vi "MIDI-Generator.vi"() -> ()   [LabVIEW 2019]
uses:
  Controls/Generator_states.ctl
panel:
  in  "Clear":bool
  in  "Save":bool
  in  "Name of message":string
  out "MIDI Events":string
  in  "Last Nibble":u16(ring)
  out "Databyte 2":i8 format="%.0x"
  out "Databyte 1":i8 format="%.0x"
  in  "Spec Concatenate":bool
  out "MIDI Event":string
  in  "Databyte 2":u16(ring) caption="Pressure" items=["0", "1", "2", "3", "4", "5", "6", "7", "8", "9", "10", "11", "12", "13", "14", "15", "16", "17", "18", "19", "20", "21", "22", "23", "24", "25", "26", "27", "28", "29", "30", "31", "32", "33", "34", "35", "36", "37", "38", "39", "40", "41", "42", "43", "44", "45", "46", "47", "48", "49", "50", "51", "52", "53", "54", "55", "56", "57", "58", "59", "60", "61", "62", "63", "64", "65", "66", "67", "68", "69", "70", "71", "72", "73", "74", "75", "76", "77", "78", "79", "80", "81", "82", "83", "84", "85", "86", "87", "88", "89", "90", "91", "92", "93", "94", "95", "96", "97", "98", "99", "100", "101", "102", "103", "104", "105", "106", "107", "108", "109", "110", "111", "112", "113", "114", "115", "116", "117", "118", "119", "120", "121", "122", "123", "124", "125", "126", "127"]
  in  "Databyte 1":u16(ring) caption="Note #" items=["C-1", "C#-1", "D-1", "D#-1", "E-1", "F-1", "F#-1", "G-1", "G#-1", "A-1", "A#-1", "B-1", "C0", "C#0", "D0", "D#0", "E0", "F0", "F#0", "G0", "G#0", "A0", "A#0", "B0", "C1", "C#1", "D1", "D#1", "E1", "F1", "F#1", "G1", "G#1", "A1", "A#1", "B1", "C2", "C#2", "D2", "D#2", "E2", "F2", "F#2", "G2", "G#2", "A2", "A#2", "B2", "C3", "C#3", "D3", "D#3", "E3", "F3", "F#3", "G3", "G#3", "A3", "A#3", "B3", "C4", "C#4", "D4", "D#4", "E4", "F4", "F#4", "G4", "G#4", "A4", "A#4", "B4", "C5", "C#5", "D5", "D#5", "E5", "F5", "F#5", "G5", "G#5", "A5", "A#5", "B5", "C6", "C#6", "D6", "D#6", "E6", "F6", "F#6", "G6", "G#6", "A6", "A#6", "B6", "C7", "C#7", "D7", "D#7", "E7", "F7", "F#7", "G7", "G#7", "A7", "A#7", "B7", "C8", "C#8", "D8", "D#8", "E8", "F8", "F#8", "G8", "G#8", "A8", "A#8", "B8", "C9", "C#9", "D9", "D#9", "E9", "F9", "F#9", "G9"]
  in  "2. Nibble":u8(ring) caption="Channel" items=["Channel 1", "Channel 2", "Channel 3", "Channel 4", "Channel 5", "Channel 6", "Channel 7", "Channel 8", "Channel 9", "Channel 10", "Channel 11", "Channel 12", "Channel 13", "Channel 14", "Channel 15", "Channel 16"]
  out "Statusbyte":i8 format="%.0x"
  in  "Status":T1(ring)
  # "Spec Concatenation"
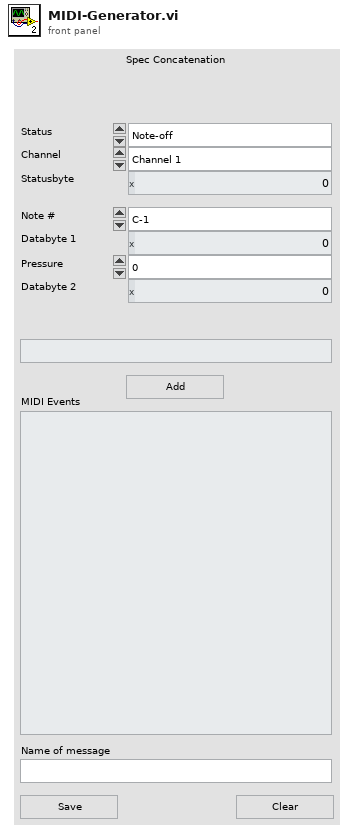
[diagram p1: front panel]
types:
  T1 = enum16{"Note-off", "Note-on", "Polyphonic Key Pressure (aftertouch)", "Control Change", "Program Change", "Channel Pressure (After-Touch)", "Pitch Bend Change", "System Common msg"}
  T2 = typedef "Generator_states.ctl" = enum16{"Initiate", "Wait for event", "Prep 2nd Nibble", "Prep Databyte 1", "Parse Databyte 1", "Prep Databyte 2", "Parse Databyte 2", "Print Event", "Save MIDI Event", "Generate Function", "Save as Textfile"}
  T3 = cluster{"1st Nibble":enum16{"Note-off", "Note-on", "Polyphonic Key Pressure (aftertouch)", "Control Change", "Program Change", "Channel Pressure (After-Touch)", "Pitch Bend Change", "System Common msg"}, "Next state":T2, "2nd Nibble":u8, "Databyte 1":u16, "Keep 2nd Nibble":bool, "Databyte 2":i32, "Last Nibble":u16, "MIDI Event":string, "MIDI Events":string}
  T4 = enum16{"open", "replace", "create", "open or create", "replace or create", "replace or create with confirmation"}
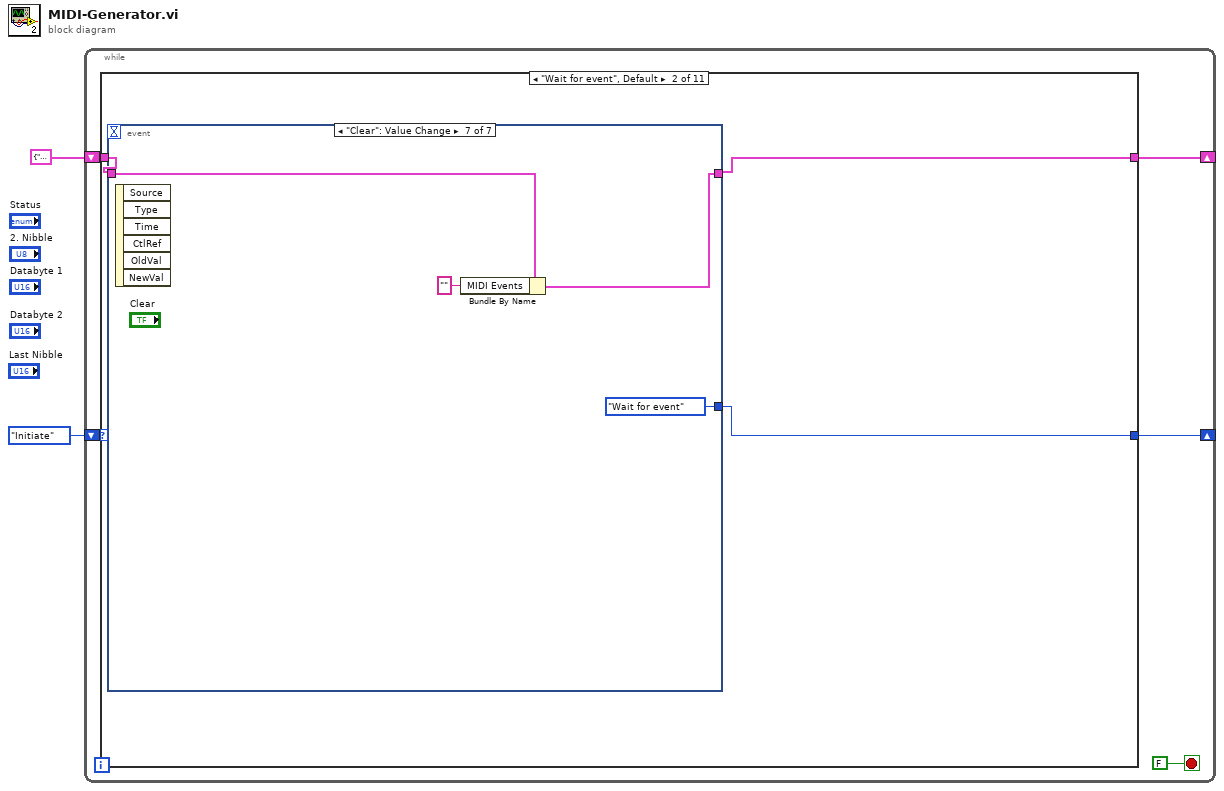
[diagram p0: block diagram]
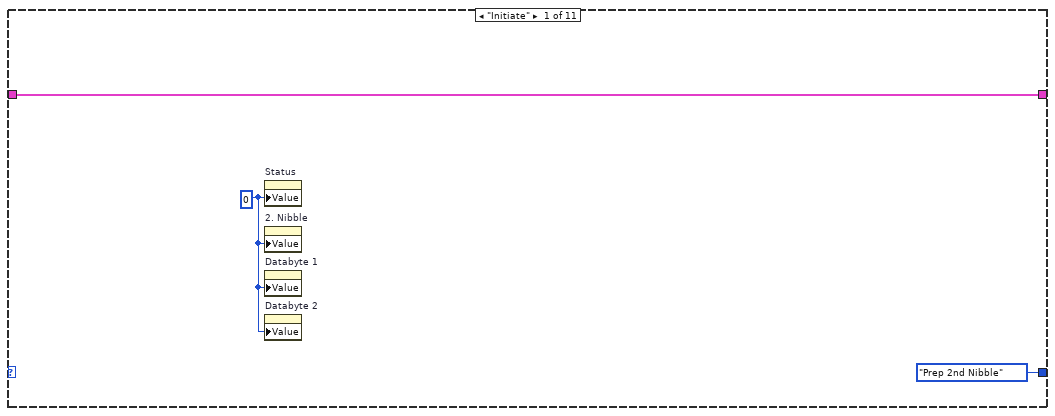
[diagram p2: hidden frame]
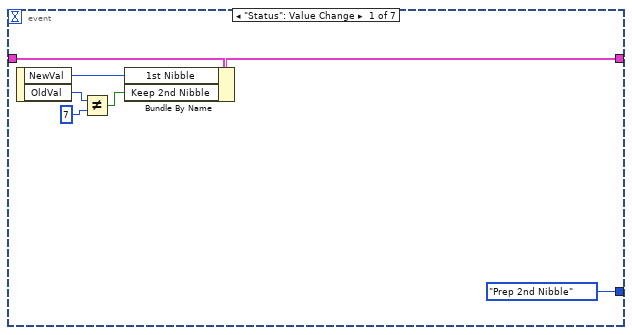
[diagram p3: hidden frame]
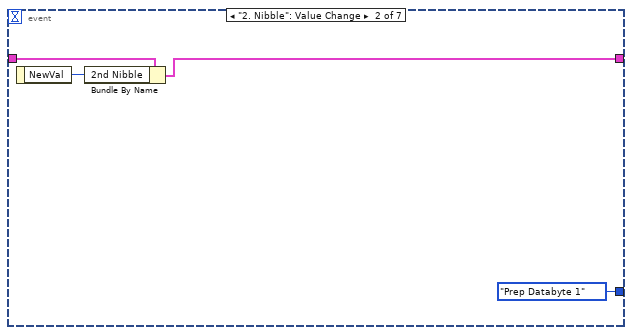
[diagram p4: hidden frame]
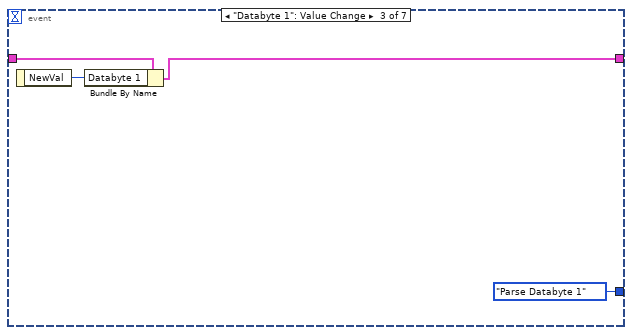
[diagram p5: hidden frame]
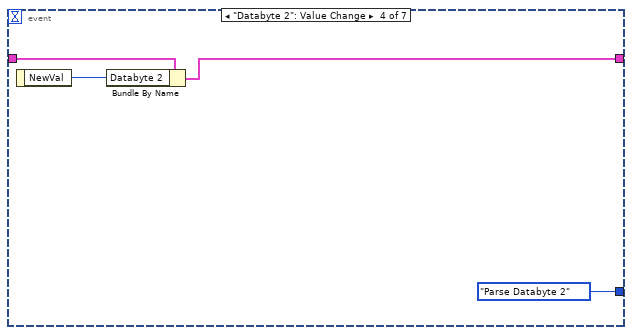
[diagram p6: hidden frame]
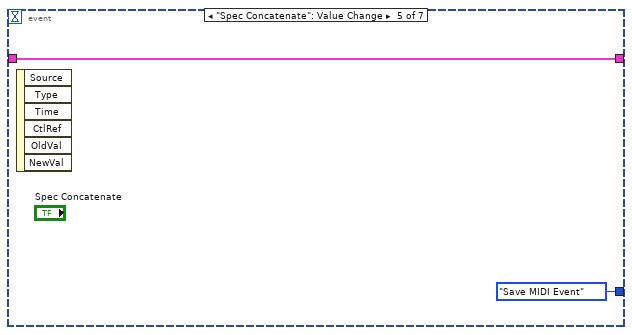
[diagram p7: hidden frame]
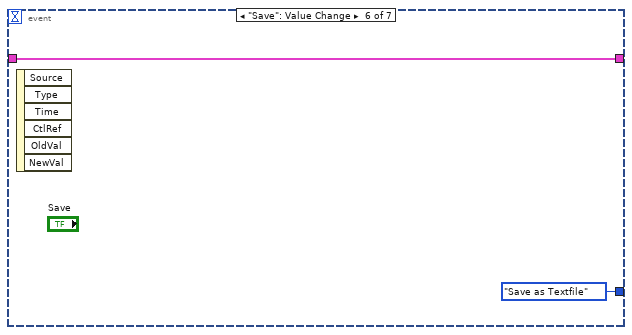
[diagram p8: hidden frame]
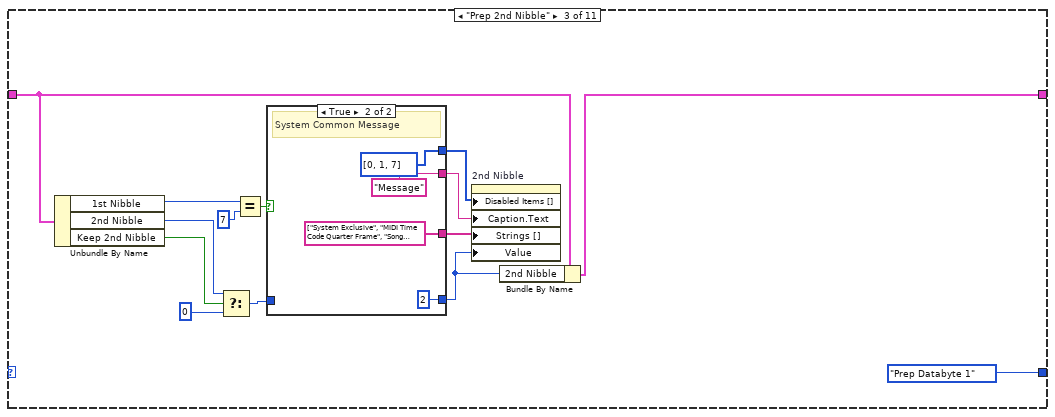
[diagram p9: hidden frame]
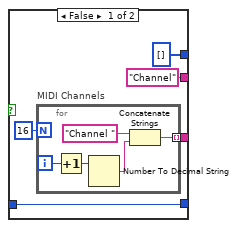
[diagram p10: hidden frame]
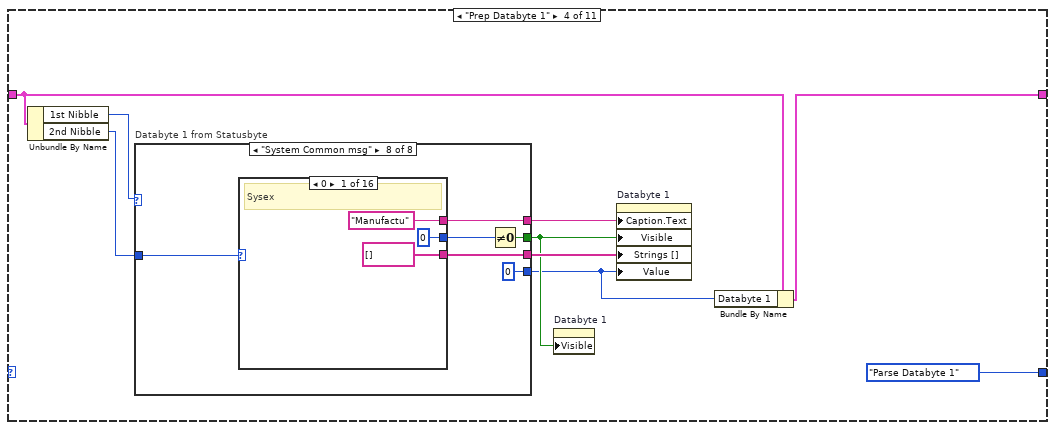
[diagram p11: hidden frame]
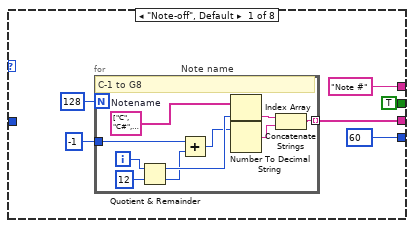
[diagram p12: hidden frame]
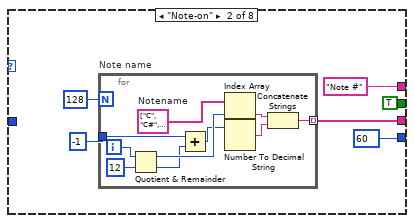
[diagram p13: hidden frame]
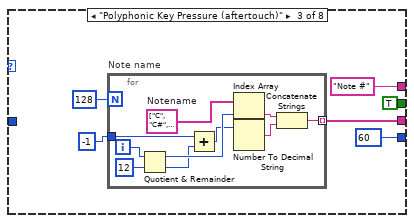
[diagram p14: hidden frame]
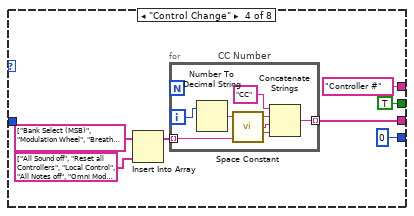
[diagram p15: hidden frame]
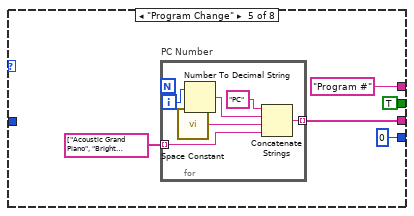
[diagram p16: hidden frame]
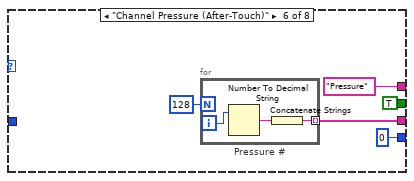
[diagram p17: hidden frame]
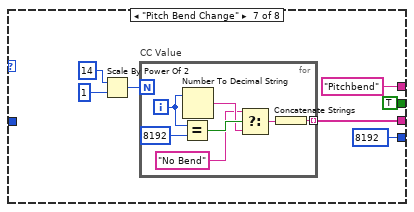
[diagram p18: hidden frame]
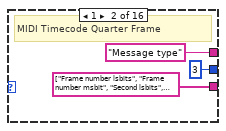
[diagram p19: hidden frame]
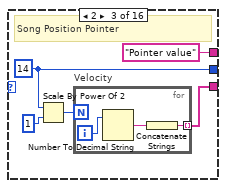
[diagram p20: hidden frame]
diagram:
  n1 = while {
    shift-right: [w3] -> _
    shift-left: T3 {"1st Nibble"=enum."Note-off", "Next state"=enum."Wait for event", "2nd Nibble"=0, "Databyte 1"=0, "Keep 2nd Nibble"=TRUE, "Databyte 2"=241, "Last Nibble"=0, "MIDI Event"="", "MIDI Events"=""} -> [w7]
    shift-right: [w4] -> _
    shift-left: Generator_states."Initiate" ("Status 2") -> [w6]
    stop <- FALSE stop-if-true
    n2 = case shown="\"Wait for event\", Default" w6 {
      tunnel: w7 -> [w10 w13 w43 w71 w239 w290 w566 w603 w621 w625 w636]
      tunnel: [w10 w12 w41 w70 w238 w288 w564 w602 w619 w625 w636] -> w3
      tunnel: [Generator_states."Prep 2nd Nibble" ("Status 2") w11 Generator_states."Prep Databyte 1" ("Status 2") Generator_states."Parse Databyte 1" ("Status 2") Generator_states."Prep Databyte 2" ("Status 2") Generator_states."Parse Databyte 2" ("Status 2") Generator_states."Print Event" ("Status 2") Generator_states."Wait for event" ("Status 2") Generator_states."Wait for event" ("Status 2") Generator_states."Wait for event" ("Status 2") Generator_states."Wait for event" ("Status 2")] -> w4
      frame "Initiate" {
        w9 = 0
        n3 = property on="Status" class="Enum (strict)"("Value"=w9) -> ()  [unwired: 2 in, 2 out]
        n4 = property on="2. Nibble" class="Ring (strict)"("Value"=w9) -> ()  [unwired: 2 in, 2 out]
        n5 = property on="Databyte 1" class="Ring (strict)"("Value"=w9) -> ()  [unwired: 2 in, 2 out]
        n6 = property on="Databyte 2" class="Ring (strict)"("Value"=w9) -> ()  [unwired: 2 in, 2 out]
      }
      frame "Wait for event", Default {
        n7 = event shown="[6] \"Clear\": Value Change" {
          selector: _ -> [_ _ _ _ _ _ _]
          dyn-events: _ -> [_ _ _ _ _ _ _]
          timeout: _ -> [_ _ _ _ _ _ _]
          tunnel: [w18 w21 w25 w30 w34 w36 w39] -> w12
          tunnel: w13 -> [w20 w23 w26 w31 w34 w36 w40]
          tunnel: [Generator_states."Prep 2nd Nibble" ("Status 2") Generator_states."Prep Databyte 1" ("Status 2") Generator_states."Parse Databyte 1" ("Status 2") Generator_states."Parse Databyte 2" ("Status 2") Generator_states."Save MIDI Event" ("Status 2") Generator_states."Save as Textfile" ("Status 2") Generator_states."Wait for event" ("Status 2")] -> w11
          event "Status": Value Change {
            n8 = event-data() -> ("NewVal"=w19:T1, "OldVal"=w16:T1)  [unwired: 1 in]
            n9 = Not Equal?(x=w16, y=7) -> (x != y?=w14:bool)
            n10 = Bundle By Name(cluster=w20, "1st Nibble"=w19, "Keep 2nd Nibble"=w14) -> (w18:T3)
          }
          event "2. Nibble": Value Change {
            n11 = event-data() -> ("NewVal"=w22:u8)  [unwired: 1 in]
            n12 = Bundle By Name(cluster=w23, "2nd Nibble"=w22) -> (w21:T3)
          }
          event "Databyte 1": Value Change {
            n13 = event-data() -> ("NewVal"=w27:u16)  [unwired: 1 in]
            n14 = Bundle By Name(cluster=w26, "Databyte 1"=w27) -> (w25:T3)
          }
          event "Databyte 2": Value Change {
            n15 = event-data() -> ("NewVal"=w32:u16)  [unwired: 1 in]
            n16 = Bundle By Name(cluster=w31, "Databyte 2"=w32) -> (w30:T3)
          }
          event "Spec Concatenate": Value Change {
            n17 = event-data() -> ()  [unwired: 1 in, 6 out]
          }
          event "Save": Value Change {
            n18 = event-data() -> ()  [unwired: 1 in, 6 out]
          }
          event "Clear": Value Change {
            n19 = event-data() -> ()  [unwired: 1 in, 6 out]
            n20 = Bundle By Name(cluster=w40, "MIDI Events"="") -> (w39:T3)
          }
        }
      }
      frame "Prep 2nd Nibble" {
        n21 = Unbundle By Name(w43) -> ("1st Nibble"=w49:T1, "2nd Nibble"=w46:u8, "Keep 2nd Nibble"=w47:bool)
        n22 = Select(t=w46, s=w47, f=u8 0) -> (s? t:f=w45:u8)
        n23 = Equal?(x=w49, y=7) -> (x = y?=w54:bool)
        n24 = case shown="True" w54 {
          tunnel: [w58 string[] ["System Exclusive", "MIDI Time Code Quarter Frame", "Song Position Pointer", "Song Select", "Undefined (Reserved) 1", "Undefined (Reserved) 2", "Tune Request", "End of Exclusive", "Timing Clock", "Undefined (Reserved) 3", "Start", "Continue", "Stop", "Undefined (Reserved) 4", "Active Sensing", "Reset"] ("System Common Messages")] -> w51
          tunnel: ["Channel" "Message" ("t")] -> w52
          tunnel: [i32[] [] ("Disabled Items []") i32[] [0, 1, 7] ("Disabled Items []")] -> w53
          tunnel: [w55 2] -> w42
          tunnel: w45 -> [w55 _]
          frame False {
            n25 = for "MIDI Channels" {
              N: 16 -> [_]
              tunnel: [w61] -> w58 mode=indexing
              i -> [w64]
              n26 = Increment(x=w64) -> (x+1=w60:i32)
              n27 = Number To Decimal String(number=w60) -> (decimal integer string=w63:string)  [unwired: 1 in]
              n28 = Concatenate Strings("Channel " ("string"), w63) -> (w61:string)
            }
          }
          frame True {
            # "System Common Message"
          }
        }
        n29 = property on="2nd Nibble" class="Ring (strict)"("Disabled Items []"=w53, "Caption.Text"=w52, "Strings []"=w51, "Value"=w42) -> ()  [unwired: 2 in, 2 out]
        n30 = Bundle By Name(cluster=w43, "2nd Nibble"=w42) -> (w41:T3)
      }
      frame "Prep Databyte 1" {
        n31 = Unbundle By Name(w71) -> ("1st Nibble"=w74:T1, "2nd Nibble"=w73:u8)
        n32 = case "Databyte 1 from Statusbyte" shown="\"System Common msg\"" w74 {
          tunnel: ["Note #" "Note #" "Note #" "Controller #" "Program #" "Pressure" "Pitchbend" w175] -> w75
          tunnel: [w79 w95 w111 w129 w140 w152 w160 w174] -> w76
          tunnel: [TRUE TRUE TRUE TRUE TRUE TRUE TRUE w177] -> w72
          tunnel: w73 -> [_ _ _ _ _ _ _ w173]
          tunnel: [60 60 60 0 0 0 8192 0] -> w69
          frame "Note-off", Default {
            n33 = for "Note name" {
              N: 128 -> [_]
              tunnel: -1 -> [w89]
              tunnel: [w84] -> w79 mode=indexing
              i -> [w92]
              w93 = string[] ["C", "C#", "D", "D#", "E", "F", "F#", "G", "G#", "A", "A#", "B"]  # Notename
              # "C-1 to G8"
              n34 = Quotient & Remainder(x=w92, y=12) -> (x-y*floor(x/y)=w90:i32, floor(x/y)=w88:i32)
              n35 = Add(x=w89, y=w88) -> (x+y=w87:i32)
              n36 = Index Array(array=w93, index=w90) -> (element=w85:string)
              n37 = Number To Decimal String(number=w87) -> (decimal integer string=w86:string)  [unwired: 1 in]
              n38 = Concatenate Strings(w85, w86) -> (w84:string)
            }
          }
          frame "Note-on" {
            n39 = for "Note name" {
              N: 128 -> [_]
              tunnel: -1 -> [w105]
              tunnel: [w100] -> w95 mode=indexing
              i -> [w108]
              w109 = string[] ["C", "C#", "D", "D#", "E", "F", "F#", "G", "G#", "A", "A#", "B"]  # Notename
              n40 = Quotient & Remainder(x=w108, y=12) -> (x-y*floor(x/y)=w106:i32, floor(x/y)=w104:i32)
              n41 = Add(x=w105, y=w104) -> (x+y=w103:i32)
              n42 = Index Array(array=w109, index=w106) -> (element=w101:string)
              n43 = Number To Decimal String(number=w103) -> (decimal integer string=w102:string)  [unwired: 1 in]
              n44 = Concatenate Strings(w101, w102) -> (w100:string)
            }
          }
          frame "Polyphonic Key Pressure (aftertouch)" {
            n45 = for "Note name" {
              N: 128 -> [_]
              tunnel: -1 -> [w121]
              tunnel: [w116] -> w111 mode=indexing
              i -> [w124]
              w125 = string[] ["C", "C#", "D", "D#", "E", "F", "F#", "G", "G#", "A", "A#", "B"]  # Notename
              n46 = Quotient & Remainder(x=w124, y=12) -> (x-y*floor(x/y)=w122:i32, floor(x/y)=w120:i32)
              n47 = Add(x=w121, y=w120) -> (x+y=w119:i32)
              n48 = Index Array(array=w125, index=w122) -> (element=w117:string)
              n49 = Number To Decimal String(number=w119) -> (decimal integer string=w118:string)  [unwired: 1 in]
              n50 = Concatenate Strings(w117, w118) -> (w116:string)
            }
          }
          frame "Control Change" {
            n51 = Insert Into Array(array=string[] ["Bank Select (MSB)", "Modulation Wheel", "Breath controller", "Undefined", "Foot Pedal (MSB)", "Portamento Time (MSB)", "Data Entry (MSB)", "Volume (MSB)", "Balance (MSB", "Undefined", "Pan position (MSB)", "Expression (MSB)", "Effect Control 1 (MSB)", "Effect Control 2 (MSB)", "Undefined", "Undefined", "General Purpose", "General Purpose", "General Purpose", "General Purpose", "Undefined", "Undefined", "Undefined", "Undefined", "Undefined", "Undefined", "Undefined", "Undefined", "Undefined", "Undefined", "Undefined", "Undefined", "Controller 0", "Controller 1", "Controller 2", "Controller 3", "Controller 4", "Controller 5", "Controller 6", "Controller 7", "Controller 8", "Controller 9", "Controller 10", "Controller 11", "Controller 12", "Controller 13", "Controller 14", "Controller 15", "Controller 16", "Controller 17", "Controller 18", "Controller 19", "Controller 20", "Controller 21", "Controller 22", "Controller 23", "Controller 24", "Controller 25", "Controller 26", "Controller 27", "Controller 28", "Controller 29", "Controller 30", "Controller 31", "Hold Pedal (on/off)", "Portamento (on/off)", "Sostenuto Pedal (on/off)", "Soft Pedal (on/off)", "Legato Pedal (on/off)", "Hold 2 Pedal (on/off)", "Sound Variation", "Resonance (Timbre)", "Sound Release Time", "Sound Attack Time", "Frequency Cutoff (Brightness)", "Sound Control 6", "Sound Control 7", "Sound Control 8", "Sound Control 9", "Sound Control 10", "Decay or General Purpose Button 1 (on/off) Roland Tone level 1", "Hi Pass Filter Frequency or General Purpose Button 2 (on/off) Roland Tone level 2", "General Purpose Button 3 (on/off) Roland Tone level 3", "General Purpose Button 4 (on/off) Roland Tone level 4", "Portamento Amount", "Undefined", "Undefined", "Undefined", "Undefined", "Undefined", "Undefined", "Reverb Level", "Tremolo Level", "Chorus Level", "Detune Level", "Phaser Level", "Data Button increment", "Data Button decrement", "Non-registered Parameter (LSB)", "Non-registered Parameter (MSB)", "Registered Parameter (LSB)", "Registered Parameter (MSB)", "Undefined", "Undefined", "Undefined", "Undefined", "Undefined", "Undefined", "Undefined", "Undefined", "Undefined", "Undefined", "Undefined", "Undefined", "Undefined", "Undefined", "Undefined", "Undefined", "Undefined", "Undefined"], new element=string[] ["All Sound off", "Reset all Controllers", "Local Control", "All Notes off", "Omni Mode off", "Omni Mode on", "Mono Mode", "Poly Mode"]) -> (w127:string[])  [unwired: 1 in]
            n52 = for "CC Number" {
              tunnel: [w136] -> w129 mode=indexing
              tunnel: w127 -> [w133] mode=indexing
              i -> [w135]
              n53 = Number To Decimal String(number=w135) -> (decimal integer string=w138:string)  [unwired: 1 in]
              n54 = call <vilib>:"Space Constant.vi"() -> ("String"=w134:string)
              n55 = Concatenate Strings("CC" ("string"), w138, w134, w133) -> (w136:string)
            }
          }
          frame "Program Change" {
            n56 = for "PC Number" {
              tunnel: [w146] -> w140 mode=indexing
              tunnel: string[] ["Acoustic Grand Piano", "Bright Acoustic Piano", "Electric Grand Piano", "Honky-tonk Piano", "Electric Piano 1", "Electric Piano 2", "Harpsichord", "Clavinet", "Celesta", "Glockenspiel", "Music Box", "Vibraphone", "Marimba", "Xylophone", "Tubular Bells", "Dulcimer", "Drawbar Organ", "Percussive Organ", "Rock Organ", "Church Organ", "Reed Organ", "Accordion", "Harmonica", "Tango accordion", "Acoustic Guitar (nylon)", "Acoustic Guitar (steel)", "Electric Guitar (jazz)", "Electric Guitar (clean)", "Electric Guitar (muted)", "Overdriven Guitar", "Distortion Guitar", "Guitar Harmonics", "Acoustic Bass", "Electric Bass (finger)", "Electric Bass (pick)", "Fretless Bass", "Slap Bass 1", "Slap Bass 2", "Synth Bass 1", "Synth Bass 2", "Violin", "Viola", "Cello", "Contrabass", "Tremolo Strings", "Pizzicato Strings", "Orchestral Harp", "Timpani", "String Ensemble 1", "String Ensemble 2", "Synth Strings 1", "Synth Strings 2", "Choir Aahs", "Voice Oohs", "Synth Choir", "Orchestra Hit", "Trumpet", "Trombone", "Tuba", "Muted Trumpet", "French Horn", "Brass Section", "Synth Brass 1", "Synth Brass 2", "Soprano Sax", "Alto Sax", "Tenor Sax", "Baritone Sax", "Oboe", "English Horn", "Bassoon", "Clarinet", "Piccolo", "Flute", "Recorder", "Pan Flute", "Blown bottle", "Shakuhachi", "Whistle", "Ocarina", "Lead 1 (square)", "Lead 2 (sawtooth)", "Lead 3 (calliope)", "Lead 4 (chiff)", "Lead 5 (charang)", "Lead 6 (voice)", "Lead 7 (fifths)", "Lead 8 (bass + lead)", "Pad 1 (new age)", "Pad 2 (warm)", "Pad 3 (polysynth)", "Pad 4 (choir)", "Pad 5 (bowed)", "Pad 6 (metallic)", "Pad 7 (halo)", "Pad 8 (sweep)", "FX 1 (rain)", "FX 2 (soundtrack)", "FX 3 (crystal)", "FX 4 (atmosphere)", "FX 5 (brightness)", "FX 6 (goblins)", "FX 7 (echoes)", "FX 8 (sci-fi)", "Sitar", "Banjo", "Shamisen", "Koto", "Kalimba", "Bagpipe", "Fiddle", "Shanai", "Tinkle Bell", "Agogo", "Steel Drums", "Woodblock", "Taiko Drum", "Melodic Tom", "Synth Drum", "Reverse Cymbal", "Guitar Fret Noise", "Breath Noise", "Seashore", "Bird Tweet", "Telephone Ring", "Helicopter", "Applause", "Gunshot", "??"] -> [w144] mode=indexing
              i -> [w149]
              n57 = call <vilib>:"Space Constant.vi"() -> ("String"=w145:string)
              n58 = Number To Decimal String(number=w149) -> (decimal integer string=w148:string)  [unwired: 1 in]
              n59 = Concatenate Strings("PC" ("string"), w148, w145, w144) -> (w146:string)
            }
          }
          frame "Channel Pressure (After-Touch)" {
            n60 = for "Pressure #" {
              N: 128 -> [_]
              tunnel: [w156] -> w152 mode=indexing
              i -> [w155]
              n61 = Number To Decimal String(number=w155) -> (decimal integer string=w157:string)  [unwired: 1 in]
              n62 = Concatenate Strings(w157) -> (w156:string)
            }
          }
          frame "Pitch Bend Change" {
            n63 = Scale By Power Of 2(n=i16 14, x=i16 1 ("n")) -> (x*2^n=w159:i16)
            n64 = for "CC Value" {
              N: w159 -> [_]
              tunnel: [w171] -> w160 mode=indexing
              i -> [w169]
              n65 = Equal?(x=w169, y=8192) -> (x = y?=w170:bool)
              n66 = Number To Decimal String(number=w169) -> (decimal integer string=w166:string)  [unwired: 1 in]
              n67 = Select(t="No Bend", s=w170, f=w166) -> (s? t:f=w167:string)
              n68 = Concatenate Strings(w167) -> (w171:string)
            }
          }
          frame "System Common msg" {
            n69 = case shown="0" w173 {
              tunnel: ["Manufactu" "Message type" "Pointer value" "Sequence" "" "" "" "" "" "" "" "" "" "" "" ""] -> w175
              tunnel: [string[] [] string[] ["Frame number lsbits", "Frame number msbit", "Second lsbits", "Second msbits", "Minute lsbits", "Minute msbits", "Hour lsbits", "Rate and hour msbit"] w185 w193 string[] [] string[] [] string[] [] string[] [] string[] [] string[] [] string[] [] string[] [] string[] [] string[] [] string[] [] string[] []] -> w174
              tunnel: [0 3 w186 w194 0 0 0 0 0 0 0 0 0 0 0 0] -> w176
              frame 0 {
                # "Sysex"
              }
              frame 1 {
                # "MIDI Timecode Quarter Frame"
              }
              frame 2 {
                w186 = 14
                # "Song Position Pointer"
                n70 = Scale By Power Of 2(n=w186, x=1) -> (x*2^n=w184:i32)
                n71 = for "Velocity" {
                  N: w184 -> [_]
                  tunnel: [w190] -> w185 mode=indexing
                  i -> [w189]
                  n72 = Number To Decimal String(number=w189) -> (decimal integer string=w191:string)  [unwired: 1 in]
                  n73 = Concatenate Strings(w191) -> (w190:string)
                }
              }
              frame 3 {
                w194 = 7
                # "Song Select"
                n74 = Scale By Power Of 2(n=w194, x=1) -> (x*2^n=w192:i32)
                n75 = for "Velocity" {
                  N: w192 -> [_]
                  tunnel: [w198] -> w193 mode=indexing
                  i -> [w197]
                  n76 = Number To Decimal String(number=w197) -> (decimal integer string=w199:string)  [unwired: 1 in]
                  n77 = Concatenate Strings(w199) -> (w198:string)
                }
              }
              frame 4, Default {
                # "Undefined 1"
              }
              frame 5 {
                # "Undefined 2"
              }
              frame 6 {
                # "Tune Request"
              }
              frame 7 {
                # "End of Exclusive"
              }
              frame 8 {
                # "Timing Clock"
              }
              frame 9 {
                # "Undefined 3"
              }
              frame 10 {
                # "Start"
              }
              frame 11 {
                # "Continue"
              }
              frame 12 {
                # "Stop"
              }
              frame 13 {
                # "Undefined 4"
              }
              frame 14 {
                # "Active Sensing"
              }
              frame 15 {
                # "Reset"
              }
            }
            n78 = Not Equal To 0?(x=w176) -> (x != 0?=w177:bool)
          }
        }
        n79 = property on="Databyte 1" class="DigNum (strict)"("Visible"=w72) -> ()  [unwired: 2 in, 2 out]
        n80 = property on="Databyte 1" class="Ring (strict)"("Caption.Text"=w75, "Visible"=w72, "Strings []"=w76, "Value"=w69) -> ()  [unwired: 2 in, 2 out]
        n81 = Bundle By Name(cluster=w71, "Databyte 1"=w69) -> (w70:T3)
      }
      frame "Parse Databyte 1" {
        n82 = Unbundle By Name(w239) -> ("1st Nibble"=w241:T1, "2nd Nibble"=w237:u8, "Databyte 1"=w240:u16)
        n83 = case shown="\"System Common msg\"" w241 {
          tunnel: w240 -> [_ _ _ _ _ _ w252 w254]
          tunnel: w239 -> [w242 w243 w244 w245 w246 w247 w251 w257]
          tunnel: [w242 w243 w244 w245 w246 w247 w250 w256] -> w238
          tunnel: w237 -> [_ _ _ _ _ _ _ w255]
          frame "Note-off", Default {
          }
          frame "Note-on" {
          }
          frame "Polyphonic Key Pressure (aftertouch)" {
          }
          frame "Control Change" {
          }
          frame "Program Change" {
          }
          frame "Channel Pressure (After-Touch)" {
          }
          frame "Pitch Bend Change" {
            n84 = Rotate(1:w252, 2:i16 -7 ("y 2")) -> (0:w248:u16)
            n85 = Subtract(x=w252, y=w248) -> (x-y=w249:u16)
            n86 = Bundle By Name(cluster=w251, "Databyte 2"=w249, "Databyte 1"=w248) -> (w250:T3)
          }
          frame "System Common msg" {
            n87 = case shown="1" w255 {
              tunnel: w257 -> [w258 w259 w264 w268 w269 w270 w271 w272 w273 w274 w275 w276 w277 w278 w279 w280]
              tunnel: [w258 w259 w265 w267 w269 w270 w271 w272 w273 w274 w275 w276 w277 w278 w279 w280] -> w256
              tunnel: w254 -> [_ _ w262 w266 _ _ _ _ _ _ _ _ _ _ _ _]
              frame 0 {
                # "Sysex"
              }
              frame 1 {
                # "MIDI Timecode Quarter Frame"
              }
              frame 2 {
                # "Song Position Pointer"
                n88 = Rotate(1:w262, 2:i16 -7 ("y 2")) -> (0:w260:u16)
                n89 = Subtract(x=w262, y=w260) -> (x-y=w261:u16)
                n90 = Bundle By Name(cluster=w264, "Databyte 2"=w261, "Databyte 1"=w260) -> (w265:T3)
              }
              frame 3 {
                # "Song Select"
                n91 = Bundle By Name(cluster=w268, "Databyte 1"=w266) -> (w267:T3)
              }
              frame 4, Default {
                # "Undefined 1"
              }
              frame 5 {
                # "Undefined 2"
              }
              frame 6 {
                # "Tune Request"
              }
              frame 7 {
                # "End of Exclusive"
              }
              frame 8 {
                # "Timing Clock"
              }
              frame 9 {
                # "Undefined 3"
              }
              frame 10 {
                # "Start"
              }
              frame 11 {
                # "Continue"
              }
              frame 12 {
                # "Stop"
              }
              frame 13 {
                # "Undefined 4"
              }
              frame 14 {
                # "Active Sensing"
              }
              frame 15 {
                # "Reset"
              }
            }
          }
        }
      }
      frame "Prep Databyte 2" {
        n92 = Unbundle By Name(w290) -> ("1st Nibble"=w294:T1, "2nd Nibble"=w286:u8, "Databyte 1"=w285:u16)
        n93 = case "Databyte 2 from Databyte 1" shown="\"System Common msg\"" w294 {
          tunnel: ["Velocity" "Velocity" "Pressure" w339 "" "" "" w409] -> w293
          tunnel: [w301 w312 w325 w337 string[] [] string[] [] string[] [] w406] -> w292
          tunnel: [TRUE TRUE TRUE w338 FALSE FALSE FALSE w407] -> w291
          tunnel: [0 127 0 0 0 0 0 0] -> w289
          tunnel: w286 -> [_ _ _ _ _ _ _ w410]
          tunnel: w285 -> [_ _ _ w335 _ _ _ w404]
          tunnel: [FALSE FALSE FALSE FALSE FALSE FALSE FALSE w402] -> w284
          tunnel: [string[] [] string[] [] string[] [] string[] [] string[] [] string[] [] string[] [] w401] -> w283
          tunnel: ["" "" "" "" "" "" "" w400] -> w282
          tunnel: [0 0 0 0 0 0 0 0] -> w281
          frame "Note-off", Default {
            n94 = for "Velocity" {
              N: 128 -> [_]
              tunnel: [w305] -> w301 mode=indexing
              i -> [w304]
              n95 = Number To Decimal String(number=w304) -> (decimal integer string=w306:string)  [unwired: 1 in]
              n96 = Concatenate Strings(w306) -> (w305:string)
            }
          }
          frame "Note-on" {
            n97 = for "Velocity" {
              N: 128 -> [_]
              tunnel: [w317] -> w312 mode=indexing
              i -> [w316]
              n98 = Number To Decimal String(number=w316) -> (decimal integer string=w318:string)  [unwired: 1 in]
              n99 = Concatenate Strings(w318) -> (w317:string)
            }
          }
          frame "Polyphonic Key Pressure (aftertouch)" {
            n100 = for "Number" {
              N: 128 -> [_]
              tunnel: [w329] -> w325 mode=indexing
              i -> [w328]
              n101 = Number To Decimal String(number=w328) -> (decimal integer string=w330:string)  [unwired: 1 in]
              n102 = Concatenate Strings(w330) -> (w329:string)
            }
          }
          frame "Control Change" {
            n103 = case "Databyte 2 from Controller #" shown="1111110" w335 {
              tunnel: [w342 string[] [] string[] [] string[] ["Off", "On"] string[] [] string[] [] string[] [] w366 string[] []] -> w337
              tunnel: ["Value" "" "" "On/Off" "" "" "" "# Channels" ""] -> w339
              tunnel: [TRUE FALSE FALSE TRUE FALSE FALSE FALSE TRUE FALSE] -> w338
              frame 128, Default {
                n104 = for "CC Value" {
                  N: 128 -> [_]
                  tunnel: [w345] -> w342 mode=indexing
                  i -> [w344]
                  n105 = Number To Decimal String(number=w344) -> (decimal integer string=w346:string)  [unwired: 1 in]
                  n106 = Concatenate Strings(w346) -> (w345:string)
                }
              }
              frame 120 {
                # "All Sound off"
              }
              frame 121 {
                # "Reset all Controllers"
              }
              frame 122 {
                # "Local Control"
              }
              frame 123 {
                # "All notes off"
              }
              frame 124 {
                # "Omni mode"
              }
              frame 125 {
                # "Omni mode"
              }
              frame 126 {
                # "Mono Mode"
                n107 = for "Databyte 2a" {
                  N: 128 -> [_]
                  tunnel: [w370] -> w366 mode=indexing
                  i -> [w369]
                  n108 = Number To Decimal String(number=w369) -> (decimal integer string=w371:string)  [unwired: 1 in]
                  n109 = Concatenate Strings(w371) -> (w370:string)
                }
              }
              frame 127 {
              }
            }
          }
          frame "Program Change" {
            # "NO SECOND DATABYTE"
          }
          frame "Channel Pressure (After-Touch)" {
            # "NO SECOND DATABYTE"
          }
          frame "Pitch Bend Change" {
          }
          frame "System Common msg" {
            n110 = case shown="1" w410 {
              tunnel: ["" w421 "Pointer value" "Sequence" "" "" "" "" "" "" "" "" "" "" "" ""] -> w409
              tunnel: [string[] [] w427 w470 w481 string[] [] string[] [] string[] [] string[] [] string[] [] string[] [] string[] [] string[] [] string[] [] string[] [] string[] [] string[] []] -> w406
              tunnel: [0 w420 w471 w482 0 0 0 0 0 0 0 0 0 0 0 0] -> w408
              tunnel: w404 -> [_ w422 _ _ _ _ _ _ _ _ _ _ _ _ _ _]
              tunnel: [0 w419 0 0 0 0 0 0 0 0 0 0 0 0 0 0] -> w403
              tunnel: ["" w418 "" "" "" "" "" "" "" "" "" "" "" "" "" ""] -> w400
              tunnel: [string[] [] w417 string[] [] string[] [] string[] [] string[] [] string[] [] string[] [] string[] [] string[] [] string[] [] string[] [] string[] [] string[] [] string[] [] string[] []] -> w401
              frame 0 {
                # "Sysex"
              }
              frame 1 {
                # "This does not work properly, I've misunderstood the spec. A MIDI TQF message should be 32 bits long...\nF0 7F 7F 01 01 hh mm ss ff F7"
                # "MIDI Timecode Quarter Frame"
                n111 = case shown="111" w422 {
                  tunnel: [4 1 4 2 4 2 4 2] -> w420
                  tunnel: ["Frame#" "Frame#" "Second" "Second" "Minute" "Minute" "Hour" "Rate"] -> w421
                  tunnel: ["" "" "" "" "" "" "" "Hour"] -> w418
                  tunnel: [0 0 0 0 0 0 0 1] -> w419
                  frame 0, Default {
                    # "Frame number lsbits"
                  }
                  frame 1 {
                    # "Frame number msbit"
                  }
                  frame 2 {
                    # "Second lsbits"
                  }
                  frame 3 {
                    # "Second msbits"
                  }
                  frame 4 {
                    # "Minute LSB"
                  }
                  frame 5 {
                    # "Minute msbits"
                  }
                  frame 6 {
                    # "Hour lsbits"
                  }
                  frame 7 {
                    # "Rate and hour msbit"
                  }
                }
                n112 = Scale By Power Of 2(n=w419, x=1) -> (x*2^n=w424:i32)
                n113 = Scale By Power Of 2(n=w420, x=1) -> (x*2^n=w425:i32)
                n114 = for "Databyte 2b" {
                  N: w424 -> [_]
                  tunnel: [w461] -> w417 mode=indexing
                  i -> [w460]
                  n115 = Number To Decimal String(number=w460) -> (decimal integer string=w462:string)  [unwired: 1 in]
                  n116 = Concatenate Strings(w462) -> (w461:string)
                }
                n117 = for "Databyte 2" {
                  N: w425 -> [_]
                  tunnel: [w464] -> w427 mode=indexing
                  i -> [w463]
                  n118 = Number To Decimal String(number=w463) -> (decimal integer string=w465:string)  [unwired: 1 in]
                  n119 = Concatenate Strings(w465) -> (w464:string)
                }
              }
              frame 2 {
                w471 = 14
                # "Song Position Pointer"
                n120 = Scale By Power Of 2(n=w471, x=1) -> (x*2^n=w469:i32)
                n121 = for "Velocity" {
                  N: w469 -> [_]
                  tunnel: [w475] -> w470 mode=indexing
                  i -> [w474]
                  n122 = Number To Decimal String(number=w474) -> (decimal integer string=w476:string)  [unwired: 1 in]
                  n123 = Concatenate Strings(w476) -> (w475:string)
                }
              }
              frame 3 {
                w482 = 7
                # "Song Select"
                n124 = Scale By Power Of 2(n=w482, x=1) -> (x*2^n=w480:i32)
                n125 = for "Velocity" {
                  N: w480 -> [_]
                  tunnel: [w486] -> w481 mode=indexing
                  i -> [w485]
                  n126 = Number To Decimal String(number=w485) -> (decimal integer string=w487:string)  [unwired: 1 in]
                  n127 = Concatenate Strings(w487) -> (w486:string)
                }
              }
              frame 4, Default {
                # "NO SECOND DATABYTE"
                # "Undefined 1"
              }
              frame 5 {
                # "NO SECOND DATABYTE"
                # "Undefined 2"
              }
              frame 6 {
                # "NO SECOND DATABYTE"
                # "Tune Request"
              }
              frame 7 {
                # "NO SECOND DATABYTE"
                # "End of Exclusive"
              }
              frame 8 {
                # "NO SECOND DATABYTE"
                # "Timing Clock"
              }
              frame 9 {
                # "NO SECOND DATABYTE"
                # "Undefined 3"
              }
              frame 10 {
                # "NO SECOND DATABYTE"
                # "Start"
              }
              frame 11 {
                # "NO SECOND DATABYTE"
                # "Continue"
              }
              frame 12 {
                # "NO SECOND DATABYTE"
                # "Stop"
              }
              frame 13 {
                # "NO SECOND DATABYTE"
                # "Undefined 4"
              }
              frame 14 {
                # "NO SECOND DATABYTE"
                # "Active Sensing"
              }
              frame 15 {
                # "NO SECOND DATABYTE"
                # "Reset"
              }
            }
            n128 = Not Equal To 0?(x=w403) -> (x != 0?=w402:bool)
            n129 = Not Equal To 0?(x=w408) -> (x != 0?=w407:bool)
          }
        }
        n130 = property on="Last Nibble" class="Ring (strict)"("Caption.Text"=w282, "Visible"=w284, "Strings []"=w283, "Value"=w281) -> ()  [unwired: 2 in, 2 out]
        n131 = property on="Databyte 2" class="DigNum (strict)"("Visible"=w291) -> ()  [unwired: 2 in, 2 out]
        n132 = property on="Databyte 2" class="Ring (strict)"("Caption.Text"=w293, "Visible"=w291, "Strings []"=w292, "Value"=w289) -> ()  [unwired: 2 in, 2 out]
        n133 = Bundle By Name(cluster=w290, "Databyte 2"=w289, "Last Nibble"=w281) -> (w288:T3)
      }
      frame "Parse Databyte 2" {
        n134 = Unbundle By Name(w566) -> ("1st Nibble"=w567:T1, "2nd Nibble"=w560:u8, "Databyte 1"=w562:u16, "Databyte 2"=w561:i32)
        n135 = case shown="\"Control Change\"" w567 {
          tunnel: w566 -> [w569 w572 w574 w578 w593 w594 w596 w599]
          tunnel: [w569 w572 w574 w578 w593 w594 w596 w599] -> w565
          tunnel: w561 -> [w570 w571 w573 w576 _ _ w597 w598]
          tunnel: [w570 w571 w573 w575 0 ("Databyte 2") 0 ("Databyte 2") w597 w598] -> w563
          tunnel: w562 -> [_ _ _ w577 _ _ _ _]
          tunnel: w560 -> [_ _ _ _ _ _ _ _]
          frame "Note-off", Default {
          }
          frame "Note-on" {
          }
          frame "Polyphonic Key Pressure (aftertouch)" {
          }
          frame "Control Change" {
            n136 = case "Databyte 2 from Controller #" shown="10000000, Default" w577 {
              tunnel: w576 -> [w579 _ _ w586 _ _ _ w590 _]
              tunnel: [w579 0 ("Databyte 2") 0 ("Databyte 2") w582 0 ("f") 0 ("f") 0 ("f") w590 0 ("Databyte 2")] -> w575
              frame 128, Default {
              }
              frame 120 {
                # "All Sound off"
              }
              frame 121 {
                # "Reset all Controllers"
              }
              frame 122 {
                # "Local Control"
                n137 = Equal To 0?(x=w586) -> (x = 0?=w585:bool)
                n138 = Select(t=0 ("Databyte 2"), s=w585, f=127) -> (s? t:f=w582:i32)
              }
              frame 123 {
                # "All notes off"
              }
              frame 124 {
                # "Omni mode"
              }
              frame 125 {
                # "Omni mode"
              }
              frame 126 {
                # "Mono Mode"
              }
              frame 127 {
              }
            }
          }
          frame "Program Change" {
          }
          frame "Channel Pressure (After-Touch)" {
          }
          frame "Pitch Bend Change" {
          }
          frame "System Common msg" {
          }
        }
        n139 = Bundle By Name(cluster=w565, "Databyte 2"=w563) -> (w564:T3)
      }
      frame "Print Event" {
        n140 = Unbundle By Name(w603) -> ("1st Nibble"=w611:T1, "2nd Nibble"=w612:u8, "Databyte 1"=w614:u16, "Databyte 2"=w615:i32)
        "Databyte 1" <- w614
        "Databyte 2" <- w615
        n141 = Add(x=w611, y=8) -> (x+y=w610:i32)
        n142 = Multiply(x=w610, y=16) -> (x*y=w609:i32)
        n143 = Add(x=w609, y=w612) -> (x+y=w613:i32)
        "Statusbyte" <- w613
        n144 = Number To Hexadecimal String(1:i16 2 ("width (-)"), 2:w613) -> (0:w616:string)
        n145 = Number To Hexadecimal String(1:i16 2 ("width (-)"), 2:w614) -> (0:w617:string)
        n146 = Number To Hexadecimal String(1:i16 2 ("width (-)"), 2:w615) -> (0:w618:string)
        n147 = Concatenate Strings(w616, w617, w618) -> (w601:string)
        "MIDI Event" <- w601
        n148 = Bundle By Name(cluster=w603, "MIDI Event"=w601) -> (w602:T3)
      }
      frame "Save MIDI Event" {
        n149 = Unbundle By Name(w621) -> ("MIDI Events"=w623:string, "MIDI Event"=w622:string)
        n150 = Concatenate Strings(w623, w622) -> (w620:string)
        "MIDI Events" <- w620
        n151 = Bundle By Name(cluster=w621, "MIDI Events"=w620) -> (w619:T3)
      }
      frame "Generate Function" {
      }
      frame "Save as Textfile" {
        n152 = Current VI's Path() -> (path=w634:path)
        n153 = Strip Path(path=w634) -> (stripped path=w633:path)  [unwired: 1 out]
        n154 = Concatenate Strings("Name of message", ".txt" ("string")) -> (w627:string)
        n155 = Build Path(base path=w633, name or relative path="midi_messages") -> (appended path=w631:path)
        n156 = Build Path(base path=w631, name or relative path=w627) -> (appended path=w630:path)
        n157 = Unbundle By Name(w636) -> ("MIDI Events"=w635:string)
        n158 = Open/Create/Replace File(file path (use dialog)=w630, operation (0:open)=T4."replace or create with confirmation") -> (refnum out=w638:refnum<file>, error out=w641:errorcluster)  [unwired: 4 in, 1 out]
        n159 = Write to Text File(file (use dialog)=w638, text=w635, error in=w641) -> (refnum out=w639:refnum<file>, error out=w640:errorcluster)  [unwired: 1 in, 1 out]
        n160 = Close File(refnum=w639, error in=w640) -> ()  [unwired: 2 out]
      }
    }
  }
